vi "Find Red Pitaya Digitizers.vi"(4 "Find linked modules":i32=4, 6 "Timeout":i32=100, 7 "Logic tags":u16[](array[numeric])=[101, 102, 104, 105, 107, 108, 109, 111, 112, 113, 114, 152, 154, 155, 157, 158, 159, 164, 169, 153], 8 "Error In":errorcluster, 9 "End address for stand-alone":i32=119, 10 "Start address":i32=100, 11 "Subnet":string="192.168.1") -> (0 "Error Out":errorcluster, 1 "Addresses":string[](array[string]), 2 "Device names":string[](array[string]), 3 "Digitizers out":refnum<class "Red Pitaya Digitizer.lvclass">[](array[class]))   [LabVIEW 2024]
uses:
  Red Pitaya Digitizer.lvclass
  C:/GitHub/NHMFL_Core/Libraries/Instruments/Instrument Driver/Instrument Driver.lvclass
  C:/GitHub/NHMFL_Core/Libraries/Instruments/Pulse Driver/Lockin Digitizer Driver/Lockin Digitizer Driver.lvclass
  Red Pitaya Modulated Digitizer/Red Pitaya Modulated Digitizer.lvclass
  C:/GitHub/NHMFL_Core/Libraries/Red Pitaya/Red Pitaya Digitizer/Red Pitaya Digitizer.lvclass
  RP Core/Rep Pitaya I-V driver/RP I-V Driver.lvclass
  Instruments/Instrument Driver/Instrument Driver.lvclass/Instrument Driver.ctl
  Red Pitaya Digitizer.lvclass/Red Pitaya Digitizer.ctl
  RP Core/RP Instrument/RP Instrument.lvclass
panel:
  out "Logic tags":u16[](array[numeric])
  out "maximum":i32
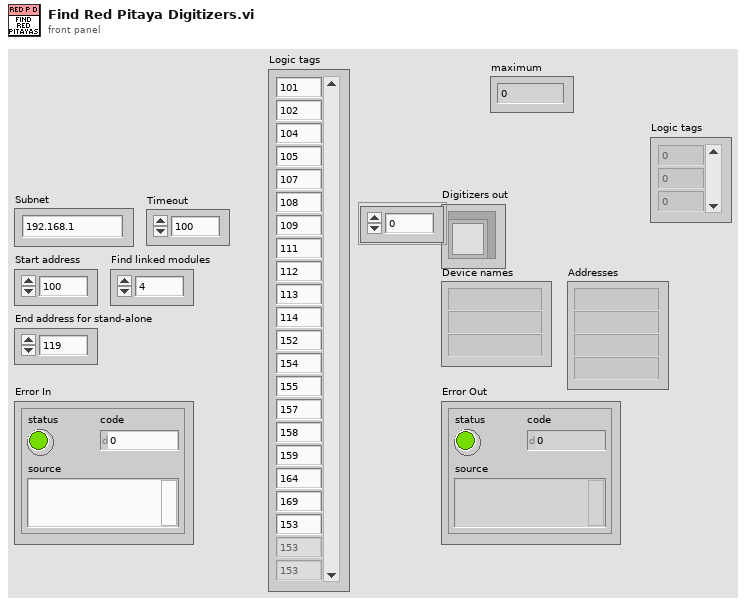
[diagram p1: front panel]
types:
  T1 = map{string, map{i32, refnum<class "RP Instrument.lvclass">}}
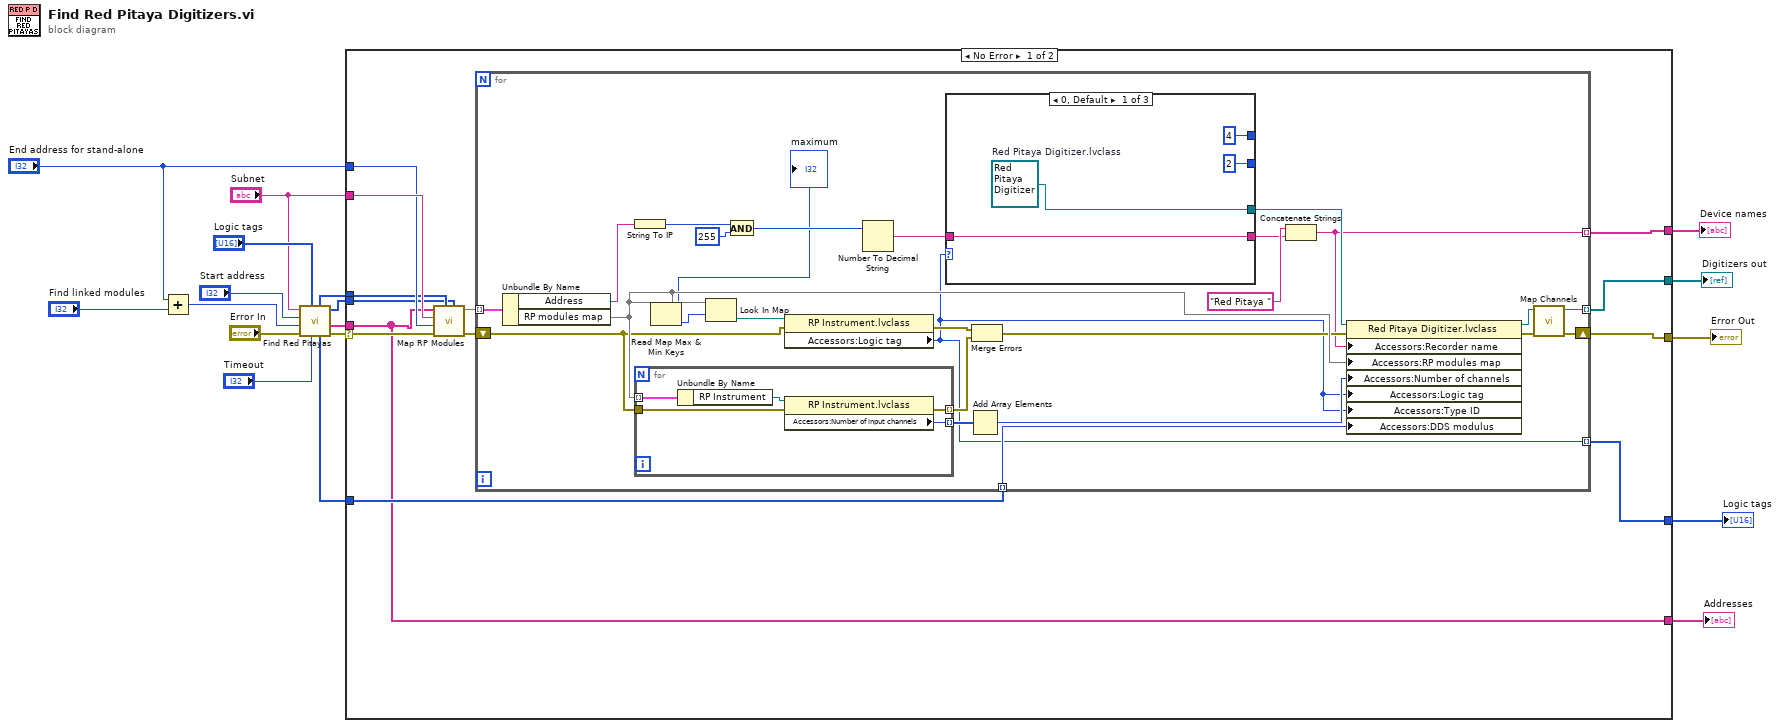
[diagram p0: block diagram]
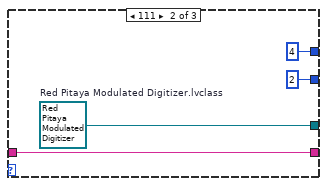
[diagram p2: hidden frame]
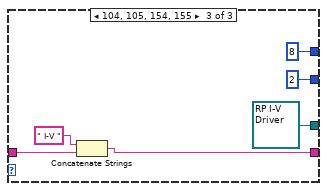
[diagram p3: hidden frame]
diagram:
  n1 = Add(x="End address for stand-alone", y="Find linked modules") -> (x+y=w14:i32)
  n2 = call "Find Red Pitayas.vi"("Timeout"="Timeout", "Logic tags"="Logic tags", "Error In"="Error In", "End address"=w14, "Start address"="Start address", "Subnet"="Subnet") -> ("Error Out"=w4:errorcluster, "Addresses"=w2:string[], "Modules"=w9:i32[], "DDS modula out"=w5:i64[], "Logic tags out"=w10:u16[])  [unwired: 1 out]
  n3 = case shown="No Error" w4 {
    selector: w4 -> [w21 w77]
    tunnel: w2 -> [w20 _]
    tunnel: "Subnet" -> [w31 _]
    tunnel: "End address for stand-alone" -> [w30 _]
    tunnel: w10 -> [w29 _]
    tunnel: w9 -> [w28 _]
    tunnel: [w25 _] -> w8
    tunnel: [w24 w77] -> w7
    tunnel: [w23 _] -> w6
    tunnel: w5 -> [w22 _]
    tunnel: [w20 _] -> w3
    tunnel: [w19 _] -> w1
    frame No Error {
      n4 = call "Map RP Modules.vi"("Modules"=w28, "Logic tags"=w29, "Error In"=w21, "End address for stand-alone"=w30, "Subnet"=w31, "Addresses"=w20) -> ("Error Out"=w26:errorcluster, "RP modules map"=w27:T1)  [unwired: 4 in]
      n5 = for {
        tunnel: w27 -> [w57] mode=indexing
        shift-right: [w36] -> w24
        shift-left: w26 -> [w43]
        tunnel: [w37] -> w25 mode=indexing
        tunnel: [w39] -> w23 mode=indexing
        tunnel: w22 -> [w33] mode=indexing
        tunnel: [w32] -> w19 mode=indexing
        n6 = Unbundle By Name(w57) -> ("Address"=w52:string, "RP modules map"=w48:map{i32, refnum<class "RP Instrument.lvclass">})
        n7 = String To IP(1:w52) -> (0:w53:u32)
        n8 = for {
          tunnel: w48 -> [w76] mode=indexing
          tunnel: [w75] -> w49 mode=indexing
          tunnel: w43 -> [w73]
          tunnel: [w72] -> w41 mode=indexing
          n9 = Unbundle By Name(w76) -> ("RP Instrument"=w74:refnum<class "RP Instrument.lvclass">)
          n10 = property class="RP Instrument.lvclass"(reference=w74, error in=w73) -> (error out=w72:errorcluster, "Accessors:Number of input channels"=w75:i32)  [unwired: 1 out]
        }
        n11 = Read Map Max & Min Keys(11:w48) -> (1:w56:i32, 3:→"maximum":i32)
        n12 = Look In Map(map=w48, key=w56) -> (value=w55:refnum<class "RP Instrument.lvclass">)  [unwired: 1 in, 1 out]
        n13 = And(x=w53, y=u32 255) -> (x .and. y?=w51:u32)
        n14 = property class="RP Instrument.lvclass"(reference=w55, error in=w43) -> (error out=w42:errorcluster, "Accessors:Logic tag"=w32:u16)  [unwired: 1 out]
        n15 = Number To Decimal String(number=w51) -> (decimal integer string=w50:string)  [unwired: 1 in]
        n16 = case shown="0, Default" w32 {
          tunnel: [w58 w65 refnum<class "RP I-V Driver.lvclass"> refnum ("RP I-V Driver.lvclass")] -> w44
          tunnel: w50 -> [w61 w64 w68]
          tunnel: [w61 w64 w70] -> w46
          tunnel: [4 ("Trigger granularity") 4 ("Trigger granularity") 8 ("Trigger granularity")] -> _
          tunnel: [2 ("Trigger granularity") 2 ("Trigger granularity") 2 ("Trigger granularity")] -> _
          frame 0, Default {
            w58 = refnum<class "Red Pitaya Digitizer.lvclass"> refnum  # Red Pitaya Digitizer.lvclass
          }
          frame 111 {
            w65 = refnum<class "Red Pitaya Modulated Digitizer.lvclass"> refnum  # Red Pitaya Modulated Digitizer.lvclass
          }
          frame 104, 105, 154, 155 {
            n17 = Concatenate Strings(" I-V " ("string"), w68) -> (w70:string)
          }
        }
        n18 = Add Array Elements(numeric array=w49) -> (sum=w45:i32)
        n19 = Merge Errors(w42, w41) -> (w40:errorcluster)
        n20 = Concatenate Strings("Red Pitaya ", w46) -> (w39:string)
        n21 = property class="Red Pitaya Digitizer.lvclass"(reference=w44, error in=w40, "Accessors:Recorder name"=w39, "Accessors:RP modules map "=w48, "Accessors:Number of channels"=w45, "Accessors:Logic tag"=w32, "Accessors:Type ID"=w32, "Accessors:DDS modulus"=w33) -> (reference out=w38:refnum<class "Red Pitaya Digitizer.lvclass">, error out=w35:errorcluster)
        n22 = call-dynamic "Map Channels.vi"("error in (no error)"=w35, "Red Pitaya Digitizer in"=w38) -> ("error out"=w36:errorcluster, "Red Pitaya Digitizer out"=w37:refnum<class "Red Pitaya Digitizer.lvclass">)  [unwired: 8 in]
      }
    }
    frame Error {
    }
  }
  "Digitizers out" <- w8
  "Device names" <- w6
  "Error Out" <- w7
  "Addresses" <- w3
  "Logic tags" <- w1
